vi "Operation Event Enable.vi"(0 "VISA resource name":refnum<visa-resource-name>, 5 "Operation Event Enable":T1, 11 "error in (no error)":errorcluster) -> (4 "VISA resource name out":refnum<visa-resource-name>, 15 "error out":errorcluster)   [LabVIEW 2012, in "NH Research Regenerative Test Series.lvlib"]
doc: "Sets the value of the Operation Enable register. This register is a mask for enabling specific bits from the Operation Event register to set the operation summary bit (OPER) of the Status Byte register. The operation summary bit is the logical OR of all enabled Operation Event register bits.\n\nThe Operation Event Enable consists of the following 15 bits:\n\nBit 0: Ready\nBit 1: Reserved\nBit 2: Ranging \nBit 3: Sweeping\nBit 4: Measuring\nBit 5: Waiting for Trigger \nBit 6: Trigger Detected\nBit 7: Reserved\nBit 8: Reserved\nBit 9: Active Mode Bit 0\nBit 10: Active Mode Bit 1\nBit 11: Active Mode Bit 2\nBit 12: Reserved\nBit 13: Reserved\nBit 14: Reserved\nBit 15: Reserved"
uses:
  <instrlib>/NH Research Regenerative Test Series/NH Research Regenerative Test Series.lvlib
panel:
  # "Bit 0:  Ready\nBit 1:  Reserved\nBit 2:  Ranging\t\nBit 3:  Sweeping\nBit 4:\t\tMeasuring\nBit 5:  Waiting for Trigger\t\nBit 6:  Trigger Detected\nBit 7:  Reserved\nBit 8:  Reserved\nBit 9:  Active Mode Bit 0\nBit 10:  Active Mode Bit 1\nBit 11:  Active Mode Bit 2\nBit 12:  Reserved\nBit 13:  Reserved\nBit 14:  Reserved\nBit 15:  Reserved"
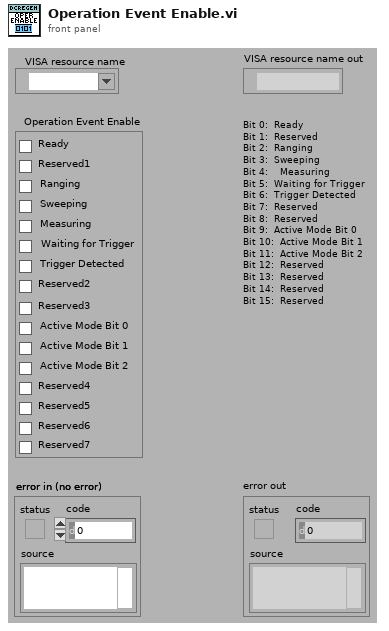
[diagram p1: front panel]
types:
  T1 = cluster{"Ready":bool, "Reserved1":bool, "Ranging":bool, "Sweeping":bool, "Measuring":bool, "Waiting for Trigger":bool, "Trigger Detected":bool, "Reserved2":bool, "Reserved3":bool, "Active Mode Bit 0":bool, "Active Mode Bit 1":bool, "Active Mode Bit 2":bool, "Reserved4":bool, "Reserved5":bool, "Reserved6":bool, "Reserved7":bool}
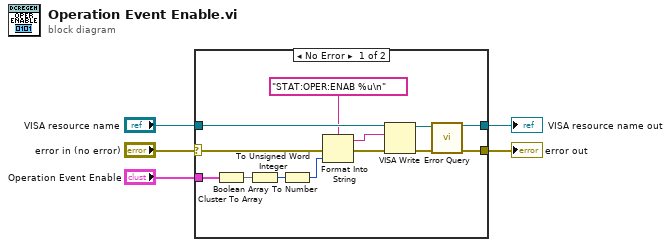
[diagram p0: block diagram]
diagram:
  n1 = case shown="No Error" "error in (no error)" {
    selector: "error in (no error)" -> [w12 w20]
    tunnel: "VISA resource name" -> [w18 w19]
    tunnel: [w16 w19] -> w5
    tunnel: [w14 w20] -> w4
    tunnel: "Operation Event Enable" -> [w8 _]
    frame No Error {
      n2 = Cluster To Array(cluster=w8) -> (array=w9:bool[])
      n3 = Boolean Array To Number(Boolean array=w9) -> (number=w7:u32)
      n4 = To Unsigned Word Integer(number=w7) -> (unsigned 16bit integer=w6:u16)
      n5 = Format Into String(format string="STAT:OPER:ENAB %u\n" ("Command to Send"), error in=w12, w6) -> (resulting string=w13:string, error out=w11:errorcluster)  [unwired: 1 in]
      n6 = VISA Write(VISA resource name=w18, write buffer=w13, error in (no error)=w11) -> (VISA resource name out=w17:refnum<visa-resource-name>, error out=w15:errorcluster)  [unwired: 1 out]
      n7 = call <instrlib>:"Error Query.vi"("VISA resource name"=w17, "error in (no error)"=w15) -> ("VISA resource name out"=w16:refnum<visa-resource-name>, "error out"=w14:errorcluster)  [unwired: 10 in, 2 out]
    }
    frame Error {
    }
  }
  "error out" <- w4
  "VISA resource name out" <- w5
